vi "LoadControlValues.vi"(8 "error in (no error)":errorcluster, 11 "path (VI name)":path) -> (0 "error out":errorcluster, 1 "file or folder exists?":bool)   [LabVIEW 2009]
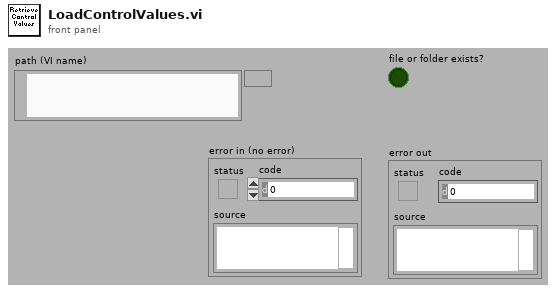
[diagram p1: front panel]
types:
  T1 = cluster{"Name":string, "type string":i16[], "data string":string}[]
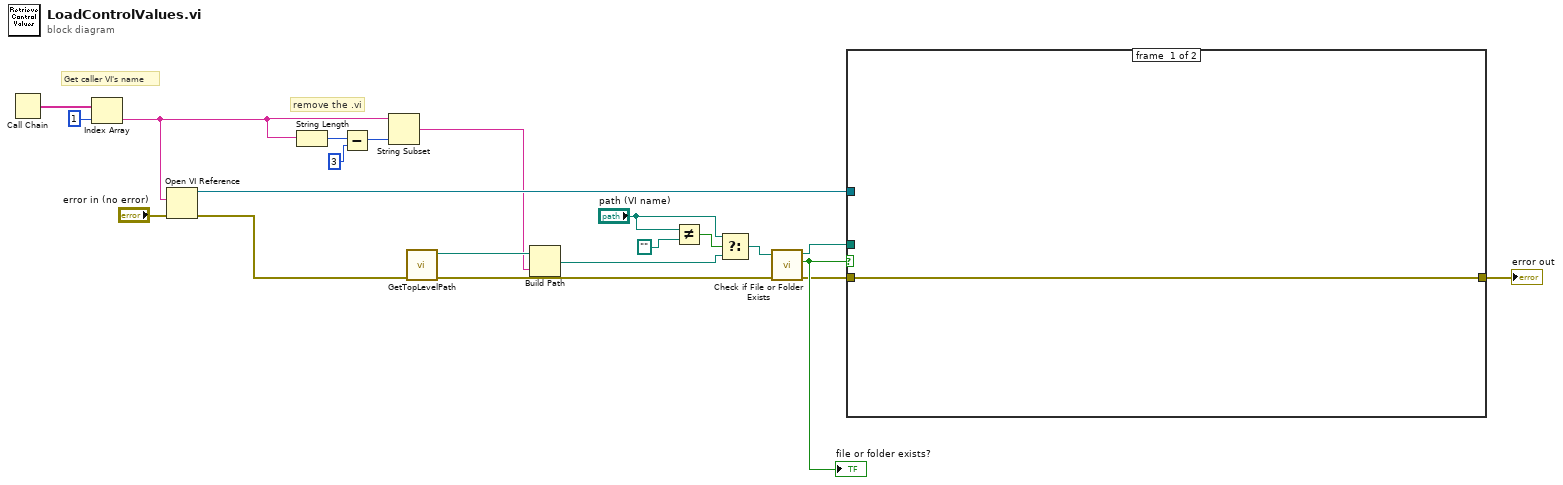
[diagram p0: block diagram]
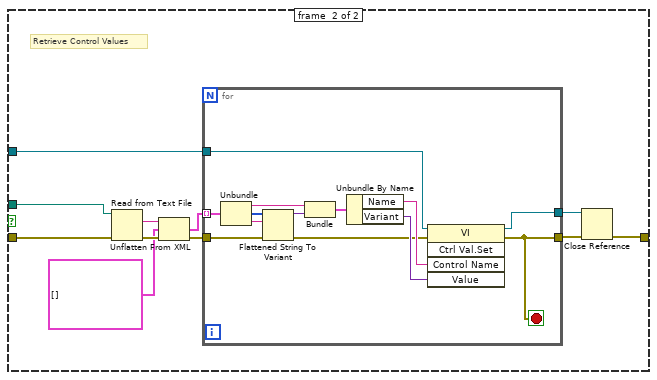
[diagram p2: hidden frame]
diagram:
  # "Get caller VI's name"
  # "remove the .vi"
  n1 = Call Chain() -> (call chain=w8:string[])
  n2 = Index Array(array=w8, index=1) -> (element=w6:string)
  n3 = Open VI Reference(vi path=w6, error in (no error)="error in (no error)") -> (vi reference=w5:refnum<vi>, error out=w4:errorcluster)  [unwired: 4 in]
  n4 = String Length(string=w6) -> (length=w16:i32)
  n5 = Subtract(x=w16, y=3) -> (x-y=w14:i32)
  n6 = String Subset(string=w6, length (rest)=w14) -> (substring=w1:string)  [unwired: 1 in]
  n7 = call "GetTopLevelPath.vi"("error in"=w4) -> ("error out"=w3:errorcluster, "path"=w2:path)  [unwired: 9 in]
  n8 = Build Path(base path=w2, name or relative path=w1) -> (appended path=w10:path)
  n9 = Not Equal?(x="path (VI name)", y=path "") -> (x != y?=w13:bool)
  n10 = Select(t="path (VI name)", s=w13, f=w10) -> (s? t:f=w9:path)
  n11 = call <vilib>:"Check if File or Folder Exists.vi"("error in (no error)"=w3, "path"=w9) -> ("error out"=w17:errorcluster, "file or folder exists?"=w19:bool, "dup path"=w20:path)  [unwired: 7 in]
  "file or folder exists?" <- w19
  n12 = case shown="False" w19 {
    tunnel: w5 -> [_ w28]
    tunnel: w20 -> [_ w27]
    tunnel: w17 -> [w22 w26]
    tunnel: [w22 w25] -> w7
    frame #0 {
    }
    frame #1 {
      # "Retrieve Control Values"
      n13 = Read from Text File(file (use dialog)=w27, error in=w26) -> (text=w33:string, error out=w31:errorcluster)  [unwired: 4 out]
      n14 = Unflatten From XML(xml string=w33, type=T1 [], error in (no error)=w31) -> (value=w29:T1, error out=w32:errorcluster)
      n15 = for {
        tunnel: w32 -> [w45]
        tunnel: [w34] -> w24
        tunnel: w29 -> [w42] mode=indexing
        tunnel: w28 -> [w36]
        tunnel: [w35] -> w23
        stop <- w34 stop-if-true
        n16 = Unbundle(w42) -> ("Name"=w43:string, "type string"=w41:i16[], "data string"=w40:string)
        n17 = Flattened String To Variant(4:w45, 6:w40, 7:w41) -> (0:w37:errorcluster, 3:w44:variant)
        n18 = Bundle("Name"=w43, "Variant"=w44) -> (w39:cluster{"Name":string, "Variant":variant})  [unwired: 1 out]
        n19 = Unbundle By Name(w39) -> ("Name"=w38:string, "Variant"=w46:variant)
        n20 = invoke class="VI" method="Ctrl Val.Set"(reference=w36, error in=w37, "Control Name"=w38, "Value"=w46) -> (reference out=w35:refnum<vi>, error out=w34:errorcluster)  [unwired: 1 in, 3 out]
      }
      n21 = Close Reference(reference=w23, error in (no error)=w24) -> (error out=w25:errorcluster)
    }
  }
  "error out" <- w7
